vi "Pre Iterate.vi"(8 "error in (no error)":errorcluster, 11 "Example Actor in":refnum<class "Example Actor.lvclass">) -> (0 "error out":errorcluster, 2 "Ready for iterations":bool, 3 "Example Actor out":refnum<class "Example Actor.lvclass">)   [LabVIEW 2023, in "Example Iterator NR Actor Implicit Iteration.lvlib" / "Example Actor.lvclass"]
doc: "Method called before the iterations"
uses:
  Example Actor.lvclass
  Example Actor.lvclass/Example Actor.ctl
  Read Ready for iterations.vi
  <userlib>/_OpenG.lib/time/time.llb/openg_time.lvlib
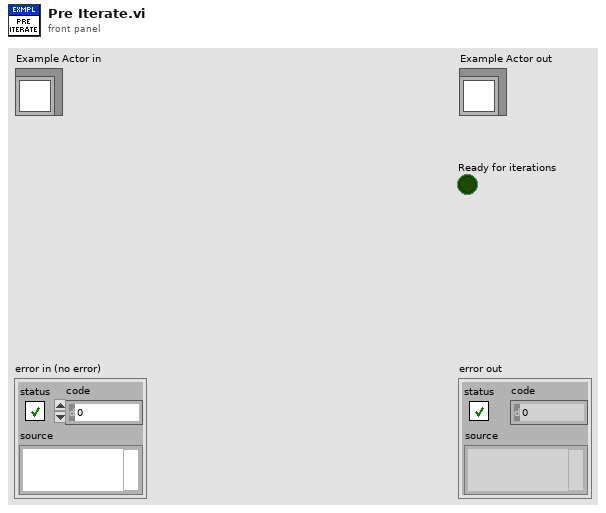
[diagram p1: front panel]
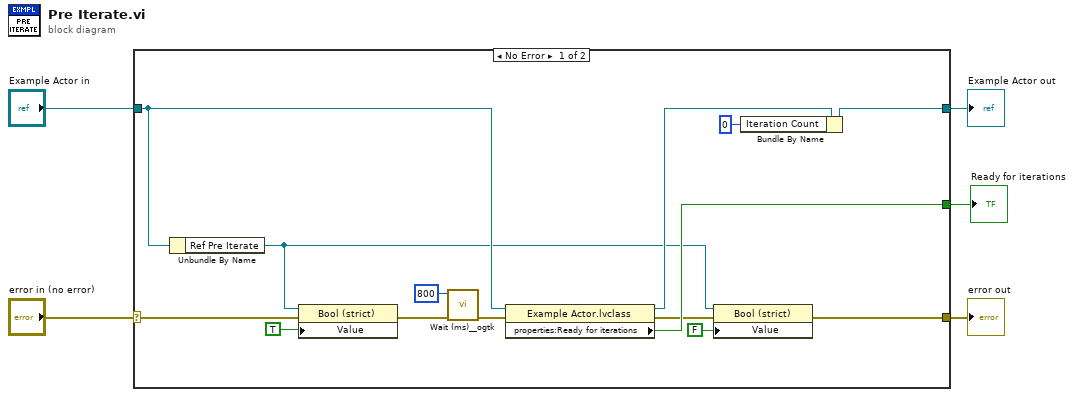
[diagram p0: block diagram]
diagram:
  n1 = case shown="No Error" "error in (no error)" {
    selector: "error in (no error)" -> [w10 w21]
    tunnel: [w8 w21] -> w4
    tunnel: [w7 w20] -> w2
    tunnel: "Example Actor in" -> [w11 w20]
    tunnel: [w16 _] -> w1
    frame No Error {
      n2 = Unbundle By Name(w11) -> ("Ref Pre Iterate"=w9:refnum<vi>)
      n3 = property class="Bool (strict)"(reference=w9, error in=w10, "Value"=TRUE) -> (error out=w13:errorcluster)  [unwired: 1 out]
      n4 = call <userlib>:"Wait (ms)__ogtk.vi"("error in (no error)"=w13, "milliseconds to wait"=u32 800) -> ("error out"=w18:errorcluster)  [unwired: 8 in, 1 out]
      n5 = property class="Example Actor.lvclass"(reference=w11, error in=w18) -> (reference out=w17:refnum<class "Example Actor.lvclass">, error out=w12:errorcluster, "properties:Ready for iterations"=w16:bool)
      n6 = property class="Bool (strict)"(reference=w9, error in=w12, "Value"=FALSE) -> (error out=w8:errorcluster)  [unwired: 1 out]
      n7 = Bundle By Name(cluster=w17, "Iteration Count"=0) -> (w7:refnum<class "Example Actor.lvclass">)
    }
    frame Error {
    }
  }
  "error out" <- w4
  "Example Actor out" <- w2
  "Ready for iterations" <- w1
